vi "Init Gesture.vi"(8 "error in (no error)":errorcluster, 11 "Grove Gesture Sensor PAJ7620U2 in":refnum<class "Grove Gesture Sensor PAJ7620U2.lvclass">) -> (0 "error out":errorcluster, 3 "Grove Gesture Sensor PAJ7620U2 out":refnum<class "Grove Gesture Sensor PAJ7620U2.lvclass">)   [LabVIEW 2020, in "CTI-Peripheral.lvlib" / "Grove Gesture Sensor PAJ7620U2.lvclass"]
uses:
  Grove Gesture Sensor PAJ7620U2.lvclass
  Grove Gesture Sensor PAJ7620U2.lvclass/Grove Gesture Sensor PAJ7620U2.ctl
  CTI/I2C Connection/I2C Connection.lvclass/I2C Connection.ctl
  CTI/Session/I2C Read Data.vi
  CTI/Session/I2C Write Data.vi
  CTI/I2C Connection/I2C Connection.lvclass
panel:
  out "Init Data":string
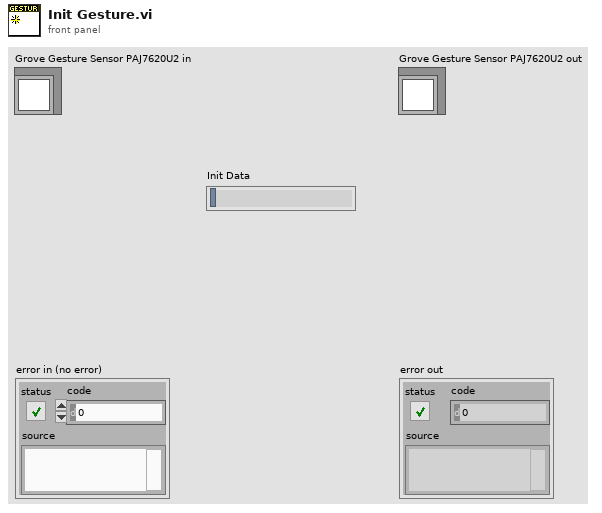
[diagram p1: front panel]
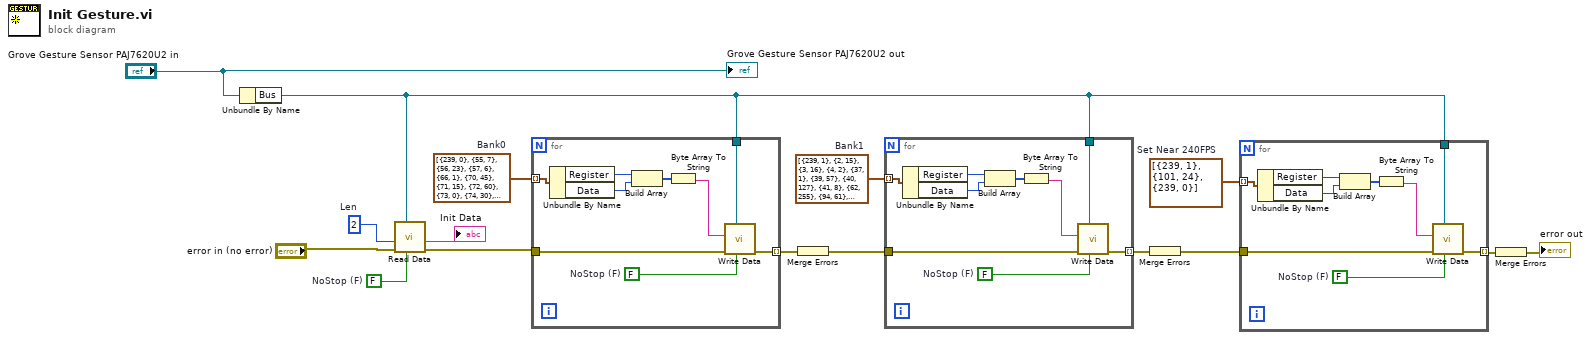
[diagram p0: block diagram]
diagram:
  w4 = FALSE  # NoStop (F)
  w6 = u8 2  # Len
  w9 = cluster{"Register":u8, "Data":u8}[] [{"Register"=239, "Data"=1}, {"Register"=101, "Data"=24}, {"Register"=239, "Data"=0}]  # Set Near 240FPS
  w12 = cluster{"Register":u8, "Data":u8}[] [{"Register"=239, "Data"=1}, {"Register"=2, "Data"=15}, {"Register"=3, "Data"=16}, {"Register"=4, "Data"=2}, {"Register"=37, "Data"=1}, {"Register"=39, "Data"=57}, {"Register"=40, "Data"=127}, {"Register"=41, "Data"=8}, {"Register"=62, "Data"=255}, {"Register"=94, "Data"=61}, {"Register"=101, "Data"=150}, {"Register"=103, "Data"=151}, {"Register"=105, "Data"=205}, {"Register"=106, "Data"=1}, {"Register"=109, "Data"=44}, {"Register"=110, "Data"=1}, {"Register"=114, "Data"=1}, {"Register"=115, "Data"=53}, {"Register"=119, "Data"=1}, {"Register"=239, "Data"=0}]  # Bank1
  w15 = cluster{"Register":u8, "Data":u8}[] [{"Register"=239, "Data"=0}, {"Register"=55, "Data"=7}, {"Register"=56, "Data"=23}, {"Register"=57, "Data"=6}, {"Register"=66, "Data"=1}, {"Register"=70, "Data"=45}, {"Register"=71, "Data"=15}, {"Register"=72, "Data"=60}, {"Register"=73, "Data"=0}, {"Register"=74, "Data"=30}, {"Register"=76, "Data"=32}, {"Register"=81, "Data"=16}, {"Register"=94, "Data"=16}, {"Register"=96, "Data"=39}, {"Register"=128, "Data"=66}, {"Register"=129, "Data"=68}, {"Register"=130, "Data"=4}, {"Register"=139, "Data"=1}, {"Register"=144, "Data"=6}, {"Register"=149, "Data"=10}, {"Register"=150, "Data"=12}, {"Register"=151, "Data"=5}, {"Register"=154, "Data"=20}, {"Register"=156, "Data"=63}, {"Register"=165, "Data"=25}, {"Register"=204, "Data"=25}, {"Register"=205, "Data"=11}, {"Register"=206, "Data"=19}, {"Register"=207, "Data"=100}, {"Register"=208, "Data"=33}]  # Bank0
  n1 = Unbundle By Name("Grove Gesture Sensor PAJ7620U2 in") -> ("Bus"=w8:refnum<class "I2C Connection.lvclass">)
  n2 = call "Read Data.vi"("NoStop (F)"=w4, "I2C Connection"=w8, "error in (no error)"="error in (no error)", "Len"=w6) -> ("error out"=w5:errorcluster, "Data"=→"Init Data":string)  [unwired: 6 in]
  n3 = for {
    tunnel: w8 -> [w24]
    tunnel: w5 -> [w22]
    tunnel: [w25] -> w14 mode=indexing
    tunnel: w15 -> [w17] mode=indexing
    w23 = FALSE  # NoStop (F)
    n4 = Unbundle By Name(w17) -> ("Register"=w20:u8, "Data"=w21:u8)
    n5 = Build Array(w20, w21) -> (w19:u8[])
    n6 = Byte Array To String(unsigned byte array=w19) -> (string=w18:string)
    n7 = call "Write Data.vi"("NoStop (F)"=w23, "I2C Connection"=w24, "error in (no error)"=w22, "Data"=w18) -> ("error out"=w25:errorcluster)  [unwired: 7 in]
  }
  n8 = Merge Errors(w14) -> (w13:errorcluster)
  n9 = for {
    tunnel: w8 -> [w33]
    tunnel: w13 -> [w31]
    tunnel: [w34] -> w11 mode=indexing
    tunnel: w12 -> [w26] mode=indexing
    w32 = FALSE  # NoStop (F)
    n10 = Unbundle By Name(w26) -> ("Register"=w29:u8, "Data"=w30:u8)
    n11 = Build Array(w29, w30) -> (w28:u8[])
    n12 = Byte Array To String(unsigned byte array=w28) -> (string=w27:string)
    n13 = call "Write Data.vi"("NoStop (F)"=w32, "I2C Connection"=w33, "error in (no error)"=w31, "Data"=w27) -> ("error out"=w34:errorcluster)  [unwired: 7 in]
  }
  n14 = Merge Errors(w11) -> (w10:errorcluster)
  n15 = for {
    tunnel: w10 -> [w41]
    tunnel: [w43] -> w2 mode=indexing
    tunnel: w9 -> [w36] mode=indexing
    tunnel: w8 -> [w35]
    w42 = FALSE  # NoStop (F)
    n16 = Unbundle By Name(w36) -> ("Register"=w39:u8, "Data"=w40:u8)
    n17 = Build Array(w39, w40) -> (w38:u8[])
    n18 = Byte Array To String(unsigned byte array=w38) -> (string=w37:string)
    n19 = call "Write Data.vi"("NoStop (F)"=w42, "I2C Connection"=w35, "error in (no error)"=w41, "Data"=w37) -> ("error out"=w43:errorcluster)  [unwired: 7 in]
  }
  n20 = Merge Errors(w2) -> (→"error out":errorcluster)
  "Grove Gesture Sensor PAJ7620U2 out" <- "Grove Gesture Sensor PAJ7620U2 in"
